vi "SubVI Open Waveform File.vi"(7 "同时播放？":bool, 8 "错误输入":errorcluster, 11 "文件路径":path) -> (0 "错误输出":errorcluster, 1 "音频输出任务ID":T1 format="%.0x", 2 "每通道采样数":i32=10000, 3 "声音文件引用句柄":T2)   [LabVIEW 2015]
uses:
  <vilib>/sound2/lvsound2.llb/Sound File Refnum.ctl
  <vilib>/sound2/lvsound2.llb/Sound Output Task ID.ctl
  <vilib>/sound2/lvsound2.llb/Sound File Info (path).vi
  <vilib>/sound2/lvsound2.llb/Sound File Read Open.vi
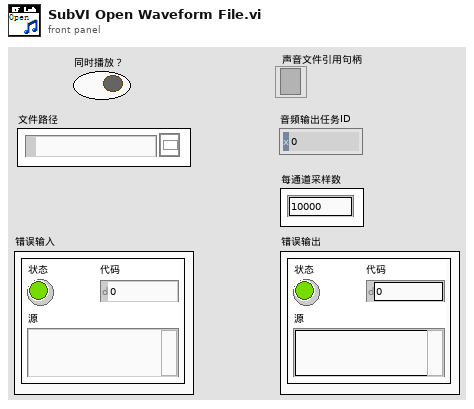
[diagram p1: front panel]
types:
  T1 = typedef "Sound Output Task ID.ctl" = u32
  T2 = typedef "Sound File Refnum.ctl" = refnum<file>
  T3 = typedef "Sound Data Format.ctl" = cluster{"sample rate (S/s)":dbl, "number of channels":i32, "bits per sample":i32}
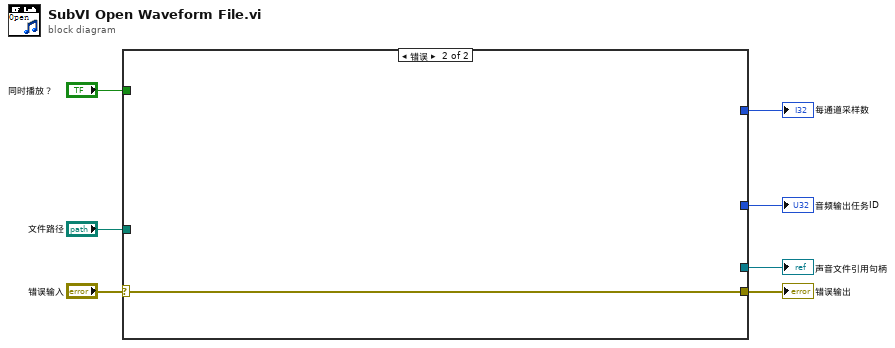
[diagram p0: block diagram]
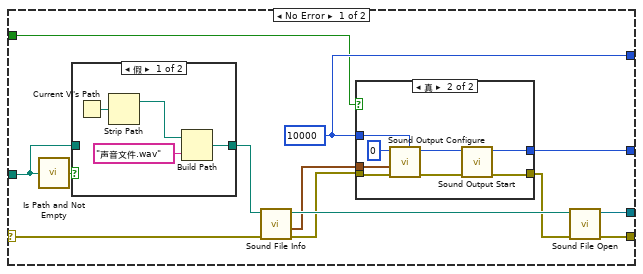
[diagram p2: hidden frame]
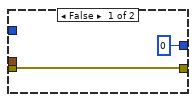
[diagram p3: hidden frame]
diagram:
  n1 = case shown="错误" "错误输入" {
    selector: "错误输入" -> [w8 w36]
    tunnel: [w20 _] -> w7
    tunnel: [w18 w36] -> w1
    tunnel: [w14 _] -> w6
    tunnel: [w13 _] -> w5
    tunnel: "文件路径" -> [w11 _]
    tunnel: "同时播放？" -> [w9 _]
    frame No Error {
      w14 = 10000 ("number of samples/ch")
      n2 = call <vilib>:"Is Path and Not Empty.vi"("path"=w11) -> ("Is Path and Not Empty?"=w12:bool)  [unwired: 4 in]
      n3 = case shown="假" w12 {
        tunnel: w11 -> [_ w35]
        tunnel: [w33 w35] -> w10
        frame False {
          n4 = Current VI's Path() -> (path=w32:path)
          n5 = Strip Path(path=w32) -> (stripped path=w31:path)  [unwired: 1 out]
          n6 = Build Path(base path=w31, name or relative path="声音文件.wav" ("名称或相对路径")) -> (appended path=w33:path)
        }
        frame True {
        }
      }
      n7 = call-poly <vilib>:"Sound File Info.vi"("error in (no error)"=w8, "path"=w10) -> ("error out"=w17:errorcluster, "sound format"=w15:T3, "path out"=w19:path)  [unwired: 6 in, 1 out]
      n8 = case shown="真" w9 {
        tunnel: w17 -> [w22 w30]
        tunnel: [w22 w28] -> w16
        tunnel: w15 -> [_ w27]
        tunnel: w14 -> [_ w25]
        tunnel: [T1 0 ("task ID out") w23] -> w13
        frame False {
        }
        frame True {
          n9 = call <vilib>:"Sound Output Configure.vi"("number of samples/ch"=w25, "error in (no error)"=w30, "sound format"=w27, "device ID"=u32 0) -> ("error out"=w29:errorcluster, "task ID"=w24:T1)  [unwired: 6 in]
          n10 = call <vilib>:"Sound Output Start.vi"("error in (no error)"=w29, "task ID"=w24) -> ("error out"=w28:errorcluster, "task ID out"=w23:T1)  [unwired: 8 in]
        }
      }
      n11 = call-poly <vilib>:"Sound File Open.vi"("error in (no error)"=w16, "path"=w19) -> ("error out"=w18:errorcluster, "sound file refnum"=w20:T2)  [unwired: 8 in]
    }
    frame Error {
    }
  }
  "错误输出" <- w1
  "声音文件引用句柄" <- w7
  "音频输出任务ID" <- w5
  "每通道采样数" <- w6
